vi "AI Read with device name.vi"(8 "error in":errorcluster, 10 "Lines":string="Dev1/port2/line0,Dev1/port2/line1,Dev1/port2/line2,Dev1/port2/line3,Dev1/port2/line4,Dev1/port2/line5,Dev1/port1/line6", 11 "Device Name":string) -> (0 "error out":errorcluster, 3 "data":dbl format="%.4f")   [LabVIEW 2013]
uses:
  <vilib>/DAQmx/create/channels.llb/DAQmx Create Channel (AI-Voltage-Basic).vi
  <vilib>/DAQmx/read.llb/DAQmx Read (Analog DBL 1Chan 1Samp).vi
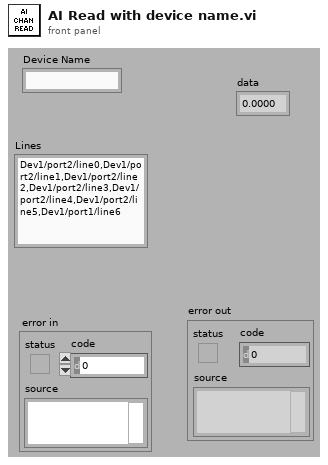
[diagram p1: front panel]
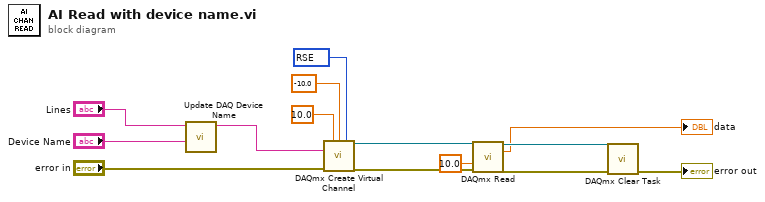
[diagram p0: block diagram]
diagram:
  w11 = 10083 items=["default"=-1, "RSE"=10083, "NRSE"=10078, "Differential"=10106, "Pseudodifferential"=12529] ("input terminal configuration")
  n1 = call "Update DAQ Device Name.vi"("Device Name"="Device Name", "Lines in (String)"="Lines") -> ("Lines out"=w1:tag)  [unwired: 9 in]
  n2 = call-poly <vilib>:"DAQmx Create Virtual Channel.vi"("maximum value"=10.0, "minimum value"=-10.0, "input terminal configuration"=w11, "physical channels"=w1, "error in"="error in") -> ("task out"=w9:refnum<k21>, "error out"=w10:errorcluster)  [unwired: 9 in]
  n3 = call-poly <vilib>:"DAQmx Read.vi"("task/channels in"=w9, "timeout"=10.0, "error in"=w10) -> ("task out"=w6:refnum<k21>, "data"=→"data":dbl, "error out"=w7:errorcluster)  [unwired: 10 in]
  n4 = call <vilib>:"DAQmx Clear Task.vi"("task in"=w6, "error in"=w7) -> ("error out"=→"error out":errorcluster)  [unwired: 13 in]
